vi "m2.vi"() -> ()   [LabVIEW 2016]
uses:
  <vilib>/rvi/interface/nirviOpenFPGA/nirviOpenFPGA.xnode
  <vilib>/rvi/interface/nirviMethod/nirviMethod.xnode
  <vilib>/FPGAPlugInAG/Dynamic/niLvFpga_Abort_Dynamic.vi
  <vilib>/FPGAPlugInAG/Dynamic/niLvFpga_Run_Dynamic.vi
  <vilib>/rvi/interface/nirviCloseFPGA/nirviCloseFPGA.xnode
  <vilib>/FPGAPlugInAG/Dynamic/niLvFpga_Reset_Dynamic.vi
  Common_RT_HealthAndStatus/RTHealthAndStatus/RTHealthAndStatus.lvclass
  MyHealthAndStatusReadFIFO/MyHealthAndStatusReadFIFO.lvclass
  MyHealthAndStatusWriteFIFO/MyHealthAndStatusWriteFIFO.lvclass
  Common_RT_Modbus/Modbus/Modbus.lvclass
  ModbusPort1ReadFIFO/ModbusPort1ReadFIFO.lvclass
  ModbusPort1WriteFIFO/ModbusPort1WriteFIFO.lvclass
  SoftwareControlledTrigger/SoftwareControlledTrigger.lvclass
  Common_RT_ILC/DataTypes/ILCSettings.ctl
  Common_RT_ILC/RTILC.lvlib
  Common_RT_ILC/ILC/ILC.lvclass
  <vilib>/rvi/interface/nirviMethod/StockFPGA_InlinedMethodWaitForSingleIRQ.vi
  <vilib>/FPGAPlugInAG/Dynamic/niLvFpga_WaitOnIrq_Dynamic.vi
  <vilib>/FPGAPlugInAG/Dynamic/niLvFpga_AcknowledgeIrq_Dynamic.vi
  Common_RT_Modbus/DynamicFrameParser/DynamicFrameParser.lvclass
  Common_RT_HPILC/HPILCFactory/HPILCFactory.lvclass
  Common_RT_HPILC/DataTypes/HPSettings.ctl
  Common_RT_HPILC/RTHPILC.lvlib
  Common_RT_HPILC/HPILC/HPILC.lvclass
  D:/Code/Common_RT_ILC/ILC/ILC.lvclass
  <vilib>/FPGAPlugInAG/Dynamic/niLvFpga_Close_Dynamic.vi
  FPGA Bitfiles/modbus1Port.lvbitx
  FPGA/main.vi
  <vilib>/FPGAPlugInAG/cRIO-9038/niLvFpga_Open_cRIO-9038.vi
  <vilib>/rvi/interface/common/dynamic/niFpgaDynamicAddResources.vi
  D:/Code/Common_RT_FPGA/IReadU32FIFO/IReadU32FIFO.lvclass
  D:/Code/Common_RT_FPGA/IReadU16FIFO/IReadU16FIFO.lvclass
  D:/Code/Common_RT_FPGA/IWriteU64FIFO/IWriteU64FIFO.lvclass
  D:/Code/Common_RT_FPGA/IWriteU16FIFO/IWriteU16FIFO.lvclass
  D:/Code/Common_RT_FPGA/IBooleanControl/IBooleanControl.lvclass
  Common_RT_ILC/DataTypes/ILCTelemetry.ctl
  Common_RT_Modbus/DataTypes/ExceptionCodes.ctl
  Common_RT_Modbus/RTModbus.lvlib
  Common_RT_ILC/DataTypes/ILCResponses.ctl
  Common_RT_HPILC/DataTypes/HPResponses.ctl
  Common_RT_HPILC/DataTypes/HPTelemetry.ctl
  Common_RT_ILC/DataTypes/ILCScanRates.ctl
panel:
  out "IRQ Timed Out 7":bool
  out "ParseSuccessful 7":bool
  in  "ForceAndStatus":bool
  out "HPTelemetry":T1
  out "HPResponses":T2 {"ForceAndStatus" items=["OK", "IllegalFunction", "IllegalDataAddress", "IllegalDataValue", "SlaveDeviceFailure", "Acknowledge", "SlaveDeviceBusy", "NegativeAcknowledge", "MemoryParityError", "GatewayPathUnavailable", "GatewayTargetDeviceFailedToRespond"]; "StepMotor" items=["OK", "IllegalFunction", "IllegalDataAddress", "IllegalDataValue", "SlaveDeviceFailure", "Acknowledge", "SlaveDeviceBusy", "NegativeAcknowledge", "MemoryParityError", "GatewayPathUnavailable", "GatewayTargetDeviceFailedToRespond"]}
  out "ParseSuccessful 6":bool
  out "IRQ Timed Out 6":bool
  in  "Steps":i8
  in  "StepMotor":bool
  in  "Boolean 2":bool
  in  "Boolean":bool
  out "IRQ Timed Out 5":bool
  out "ParseSuccessful 5":bool
  out "IRQ Timed Out 4":bool
  out "ParseSuccessful 4":bool
  out "IRQ Timed Out 3":bool
  out "ParseSuccessful 3":bool
  out "IRQ Timed Out 2":bool
  out "ParseSuccessful 2":bool
  out "ILCResponses":T4 {"ReadCalibration" items=["OK", "IllegalFunction", "IllegalDataAddress", "IllegalDataValue", "SlaveDeviceFailure", "Acknowledge", "SlaveDeviceBusy", "NegativeAcknowledge", "MemoryParityError", "GatewayPathUnavailable", "GatewayTargetDeviceFailedToRespond"]; "ReadDAC" items=["OK", "IllegalFunction", "IllegalDataAddress", "IllegalDataValue", "SlaveDeviceFailure", "Acknowledge", "SlaveDeviceBusy", "NegativeAcknowledge", "MemoryParityError", "GatewayPathUnavailable", "GatewayTargetDeviceFailedToRespond"]; "ADCOffsetSensitivity" items=["OK", "IllegalFunction", "IllegalDataAddress", "IllegalDataValue", "SlaveDeviceFailure", "Acknowledge", "SlaveDeviceBusy", "NegativeAcknowledge", "MemoryParityError", "GatewayPathUnavailable", "GatewayTargetDeviceFailedToRespond"]; "ADCScanRate" items=["OK", "IllegalFunction", "IllegalDataAddress", "IllegalDataValue", "SlaveDeviceFailure", "Acknowledge", "SlaveDeviceBusy", "NegativeAcknowledge", "MemoryParityError", "GatewayPathUnavailable", "GatewayTargetDeviceFailedToRespond"]; "Reset" items=["OK", "IllegalFunction", "IllegalDataAddress", "IllegalDataValue", "SlaveDeviceFailure", "Acknowledge", "SlaveDeviceBusy", "NegativeAcknowledge", "MemoryParityError", "GatewayPathUnavailable", "GatewayTargetDeviceFailedToRespond"]; "SetTemporaryAddress" items=["OK", "IllegalFunction", "IllegalDataAddress", "IllegalDataValue", "SlaveDeviceFailure", "Acknowledge", "SlaveDeviceBusy", "NegativeAcknowledge", "MemoryParityError", "GatewayPathUnavailable", "GatewayTargetDeviceFailedToRespond"]; "ILCMode" items=["OK", "IllegalFunction", "IllegalDataAddress", "IllegalDataValue", "SlaveDeviceFailure", "Acknowledge", "SlaveDeviceBusy", "NegativeAcknowledge", "MemoryParityError", "GatewayPathUnavailable", "GatewayTargetDeviceFailedToRespond"]; "ReportServerStatus" items=["OK", "IllegalFunction", "IllegalDataAddress", "IllegalDataValue", "SlaveDeviceFailure", "Acknowledge", "SlaveDeviceBusy", "NegativeAcknowledge", "MemoryParityError", "GatewayPathUnavailable", "GatewayTargetDeviceFailedToRespond"]; "ReportServerID" items=["OK", "IllegalFunction", "IllegalDataAddress", "IllegalDataValue", "SlaveDeviceFailure", "Acknowledge", "SlaveDeviceBusy", "NegativeAcknowledge", "MemoryParityError", "GatewayPathUnavailable", "GatewayTargetDeviceFailedToRespond"]}
  out "ParseSuccessful":bool
  out "IRQ Timed Out":bool
  out "ILCTelemetry":T5 {"ADCScanRate" items=["50 Hz"=0, "60 Hz"=1, "100 Hz"=2, "120 Hz"=3, "200 Hz"=4, "240 Hz"=5, "300 Hz"=6, "400 Hz"=7, "480 Hz"=8, "600 Hz"=9, "1200 Hz"=10, "2400 Hz"=11, "4800 Hz"=12, "No Change"=255]}
  in  "SetTemporaryAddress":bool
  in  "Reset":bool
  in  "ReportServerStatus":bool
  in  "ReportServerID":bool
  in  "TemporaryAddress":u8
  in  "ILCMode":u16
  in  "SetILCMode":bool
  out "Port 1 Status Bits":u64 format="%016b"
  out "error out":errorcluster
  out "Port 1 Frames Received":i64
  out "Port 1 Bytes Received":i64
  out "Port 1 Frames Transmitted":i64
  out "Port 1 Bytes Transmitted":i64
  # "Port 1 = Modbus"
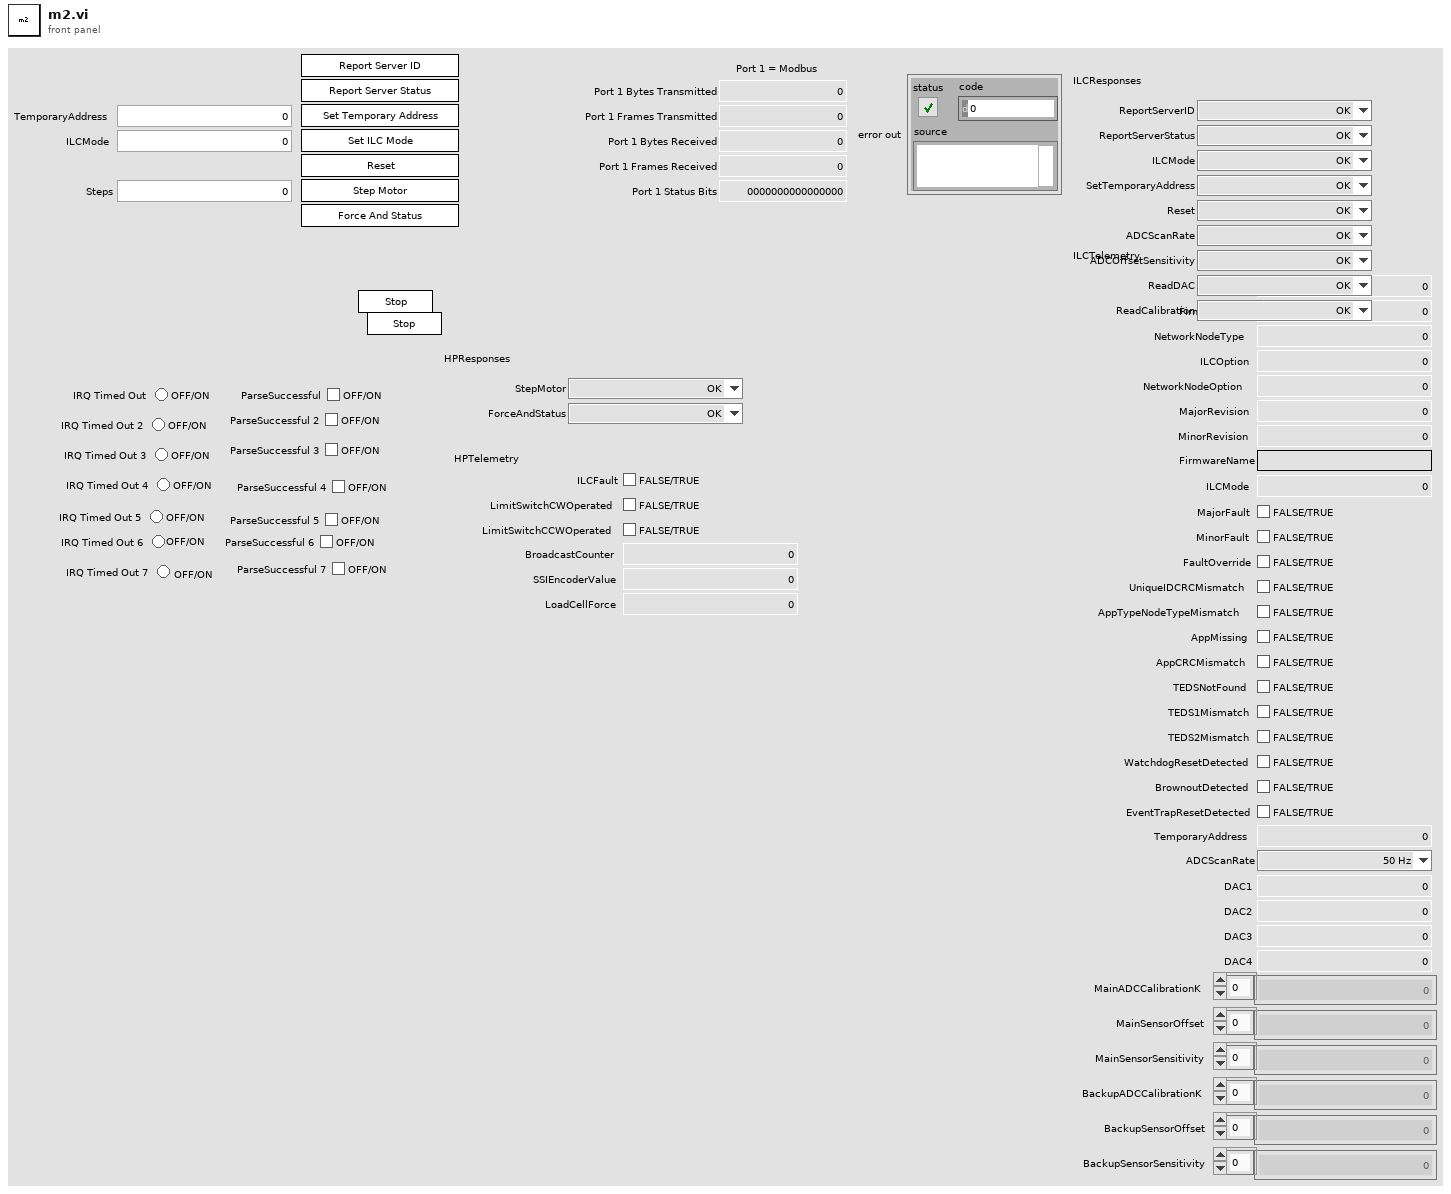
[diagram p1: front panel]
types:
  T1 = typedef "RTHPILC.lvlib/HPTelemetry.ctl" = cluster{"ILCFault":bool, "LimitSwitchCWOperated":bool, "LimitSwitchCCWOperated":bool, "BroadcastCounter":u8, "SSIEncoderValue":i32, "LoadCellForce":sgl}
  T2 = typedef "RTHPILC.lvlib/HPResponses.ctl" = cluster{"StepMotor":T3, "ForceAndStatus":T3}
  T3 = typedef "RTModbus.lvlib/ExceptionCodes.ctl" = u16
  T4 = typedef "RTILC.lvlib/ILCResponses.ctl" = cluster{"ReportServerID":T3, "ReportServerStatus":T3, "ILCMode":T3, "SetTemporaryAddress":T3, "Reset":T3, "ADCScanRate":T3, "ADCOffsetSensitivity":T3, "ReadDAC":T3, "ReadCalibration":T3}
  T5 = typedef "RTILC.lvlib/ILCTelemetry.ctl" = cluster{"UniqueID":u64, "FirmwareType":u8, "NetworkNodeType":u8, "ILCOption":u8, "NetworkNodeOption":u8, "MajorRevision":u8, "MinorRevision":u8, "FirmwareName":string, "ILCMode":u16, "MajorFault":bool, "MinorFault":bool, "FaultOverride":bool, "UniqueIDCRCMismatch":bool, "AppTypeNodeTypeMismatch":bool, "AppMissing":bool, "AppCRCMismatch":bool, "TEDSNotFound":bool, "TEDS1Mismatch":bool, "TEDS2Mismatch":bool, "WatchdogResetDetected":bool, "BrownoutDetected":bool, "EventTrapResetDetected":bool, "TemporaryAddress":u8, "ADCScanRate":T6, "DAC1":u16, "DAC2":u16, "DAC3":u16, "DAC4":u16, "MainADCCalibrationK":sgl[], "MainSensorOffset":sgl[], "MainSensorSensitivity":sgl[], "BackupADCCalibrationK":sgl[], "BackupSensorOffset":sgl[], "BackupSensorSensitivity":sgl[]}
  T6 = typedef "RTILC.lvlib/ILCScanRates.ctl" = u8
  T7 = typedef "RTHPILC.lvlib/HPSettings.ctl" = cluster{"ILCSettings":T8, "ID":i16, "ReferencePosition":i32}
  T8 = typedef "RTILC.lvlib/ILCSettings.ctl" = cluster{"Subnet":u8, "Address":u8}
  T9 = typedef "RTModbus.lvlib/Frame.ctl" = cluster{"Data":u8[], "WaitForTrigger":bool, "WaitForRx":u16, "TriggerIRQ":bool, "DelayTicks":u16, "DelayMicroseconds":u16, "DelayMilliseconds":u16}
  T10 = typedef "RTILC.lvlib/ILCData.ctl" = cluster{"Constants":T11, "Command":T12, "Telemetry":T5, "Responses":T4, "Timings":T13}
  T11 = typedef "RTILC.lvlib/ILCConstants.ctl" = cluster{"Subnet":u8, "Address":u8}
  T12 = typedef "RTILC.lvlib/ILCCommand.ctl" = cluster{"ILCMode":u16, "TemporaryAddress":u8, "ADCScanRate":T6, "ADCChannel":u8, "ADCOffset":sgl, "ADCSensitivity":sgl}
  T13 = typedef "RTILC.lvlib/ILCTimings.ctl" = cluster{"ADCOffsetSensitivity":u32, "ADCScanRate":u32, "ILCMode":u32, "ReadCalibration":u32, "ReportServerID":u32, "ReportServerStatus":u32, "Reset":u32, "SetTemporaryAddress":u32}
  T14 = typedef "RTHPILC.lvlib/HPData.ctl" = cluster{"Constants":T15, "Command":T16, "Telemetry":T1, "Responses":T2, "Timings":T17}
  T15 = typedef "RTHPILC.lvlib/HPConstants.ctl" = cluster{"ID":i16, "ReferencePosition":i32}
  T16 = typedef "RTHPILC.lvlib/HPCommand.ctl" = cluster{"Steps":i8}
  T17 = typedef "RTHPILC.lvlib/HPTimings.ctl" = cluster{"BroadcastStepMotor":u32, "ForceAndStatus":u32, "FreezeSensorValues":u32, "StepMotor":u32}
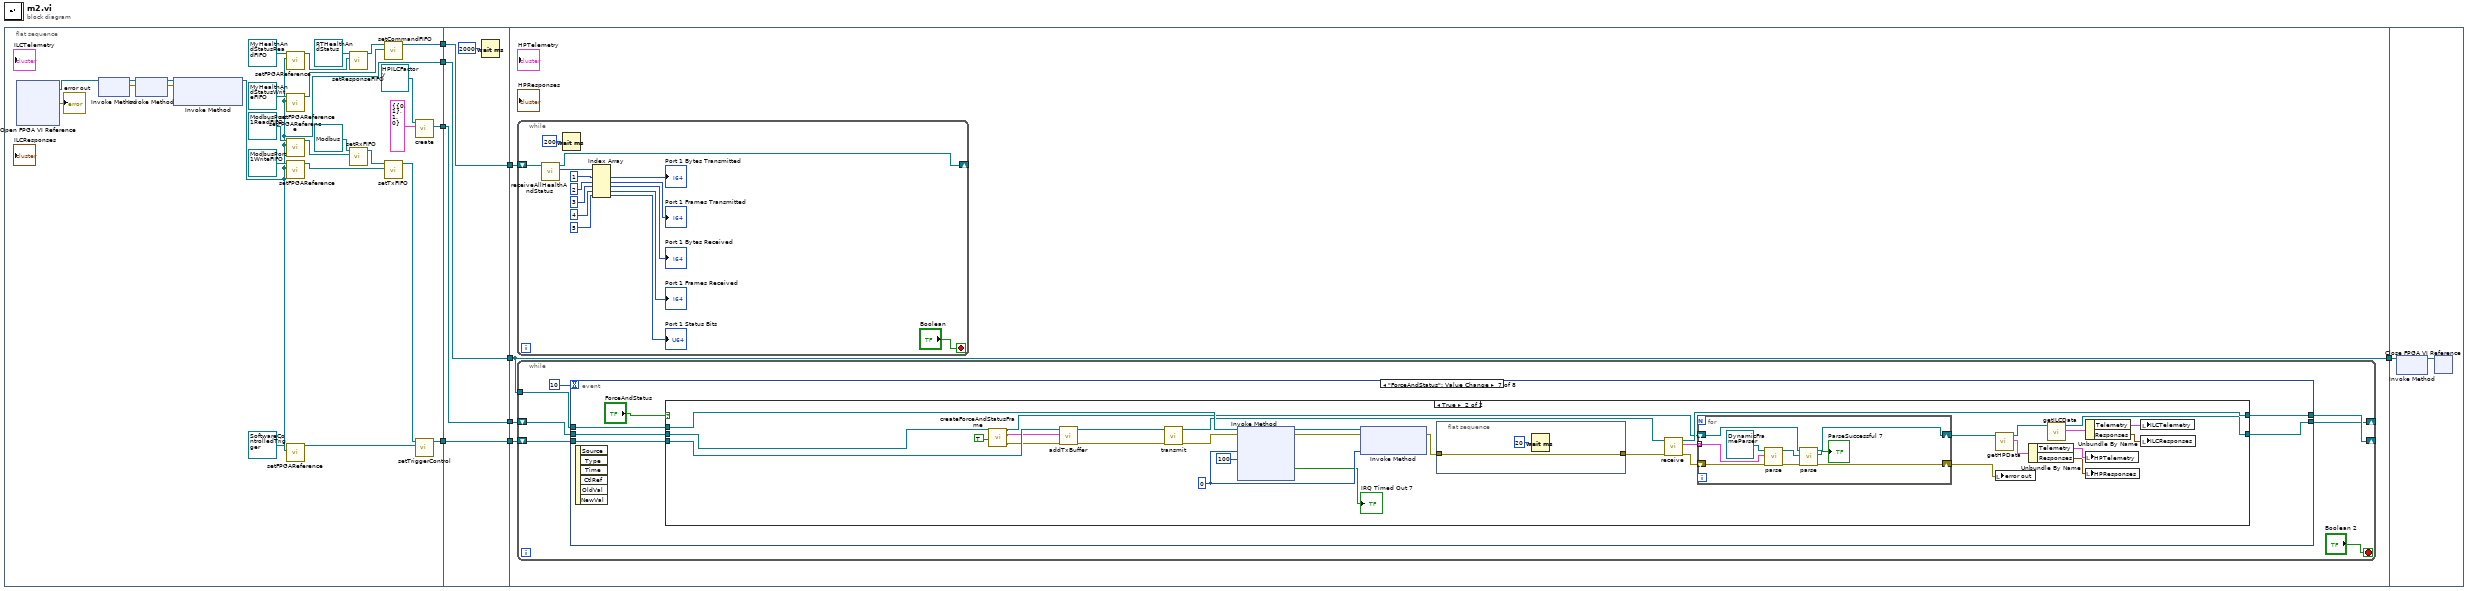
[diagram p0: block diagram]
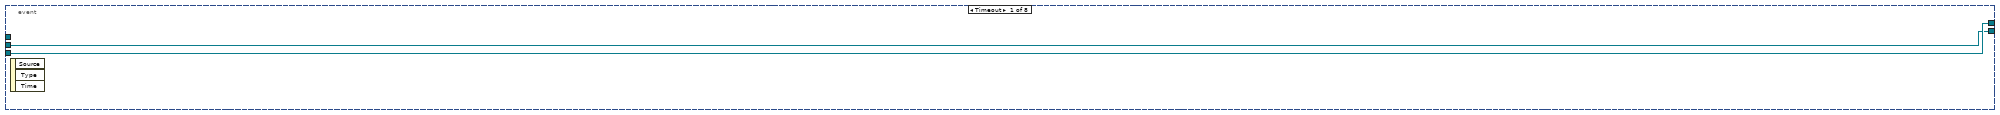
[diagram p2: hidden frame]
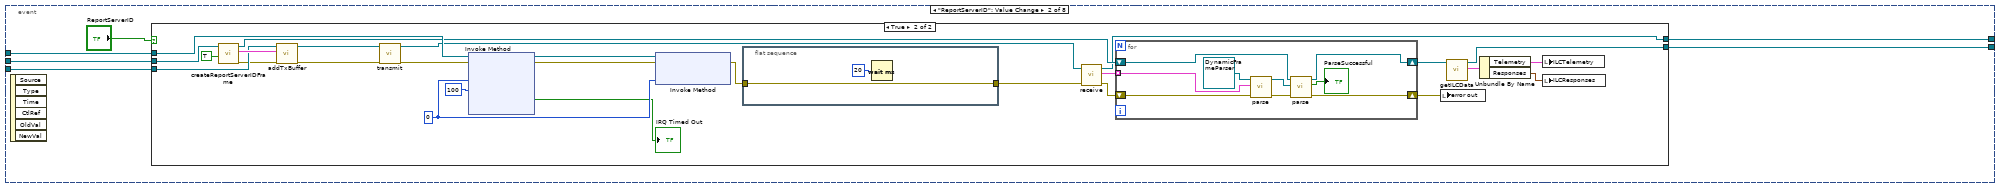
[diagram p3: hidden frame]
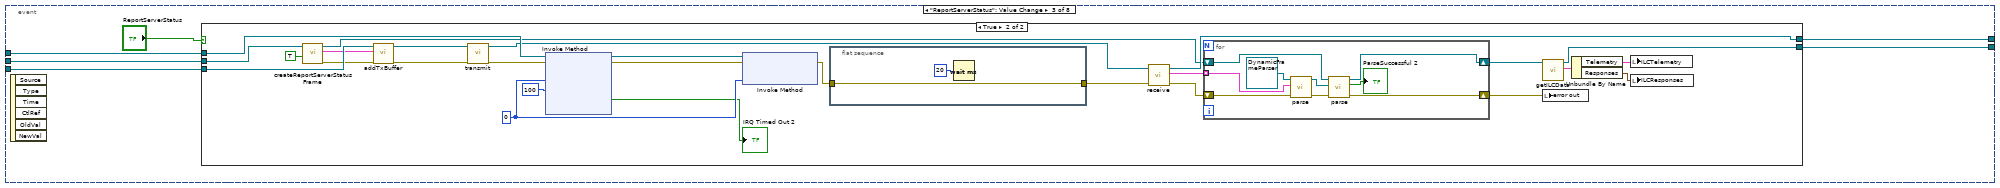
[diagram p5: hidden frame]
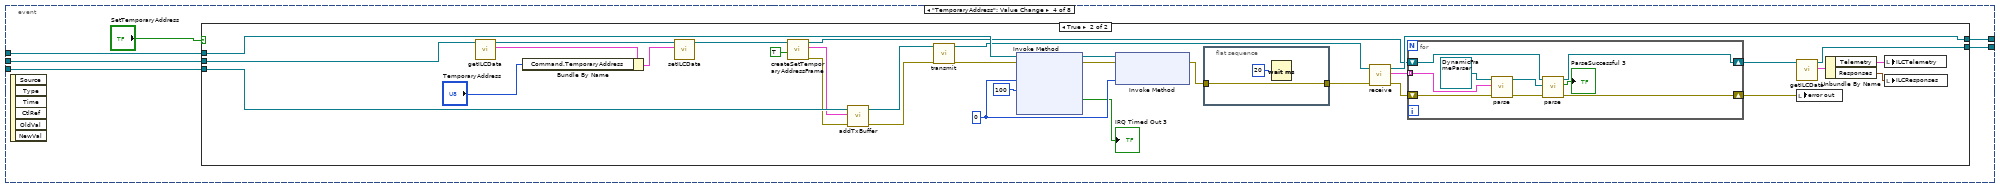
[diagram p7: hidden frame]
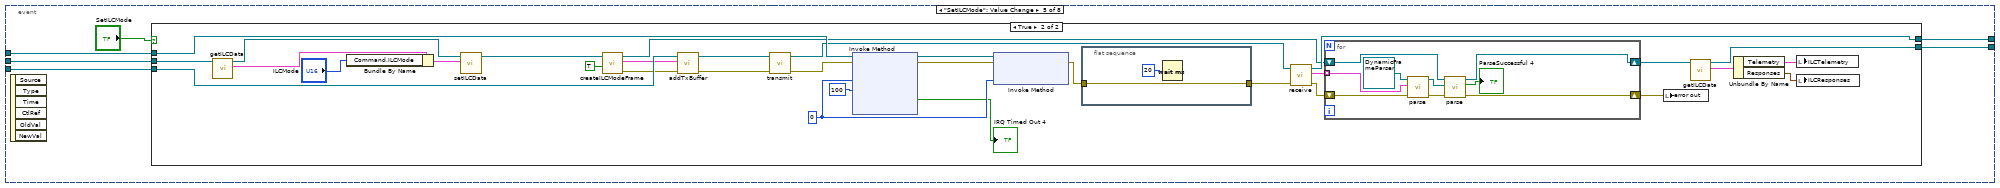
[diagram p9: hidden frame]
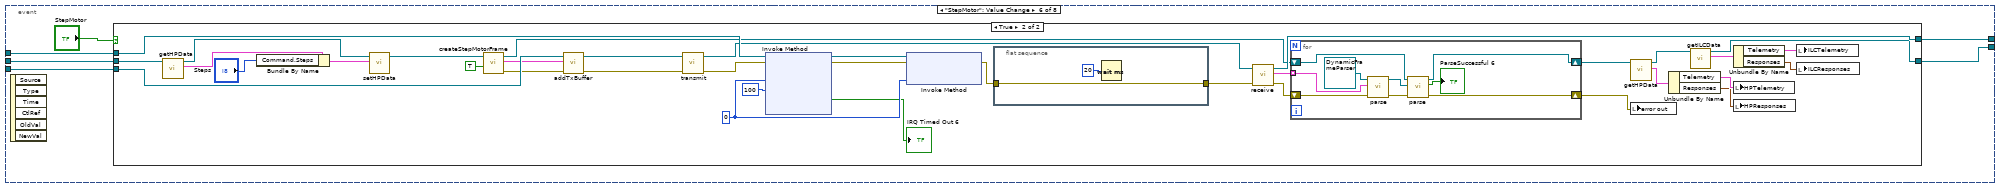
[diagram p11: hidden frame]
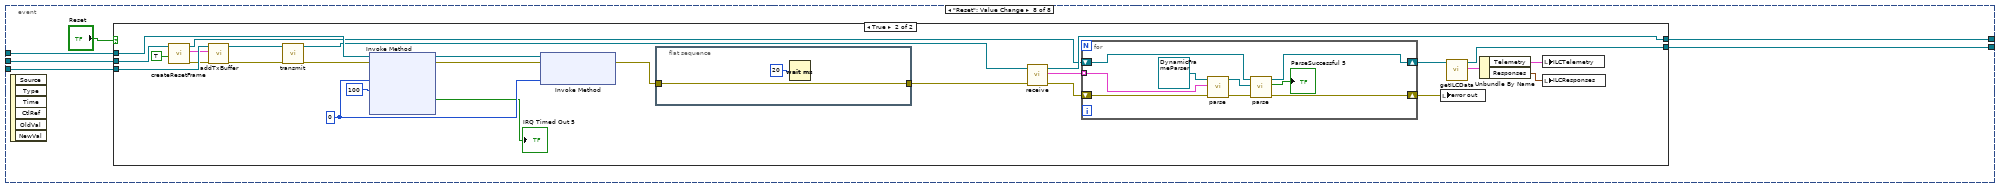
[diagram p14: hidden frame]
diagram:
  n1 = flat-sequence {
    tunnel: [w17] -> w9
    tunnel: [w14] -> w6
    tunnel: [w32] -> w4
    tunnel: [w10] -> w1
    tunnel: w9 -> [w41]
    tunnel: [w41] -> w8
    tunnel: w6 -> [w39]
    tunnel: [w39] -> w5
    tunnel: w4 -> [w38]
    tunnel: [w38] -> w3
    tunnel: [w37] -> w2
    tunnel: w1 -> [w37]
    tunnel: w8 -> [w42]
    tunnel: [w42] -> w7
    tunnel: w5 -> [w45]
    tunnel: w3 -> [w44]
    tunnel: w2 -> [w43]
    tunnel: w7 -> [w415]
    frame #0 {
      n2 = xnode "Open FPGA VI Reference"() -> ("FPGA VI Reference Out"=w19:refnum<k20>, "error out"=→"error out":errorcluster)  [unwired: 2 in]
      n3 = xnode "Invoke Method"("FPGA VI Reference In"=w19) -> ("FPGA VI Reference Out"=w36:refnum<k20>, "error out"=w21:errorcluster)  [unwired: 1 in]
      n4 = xnode "Invoke Method"("FPGA VI Reference In"=w36, "error in"=w21) -> ("FPGA VI Reference Out"=w35:refnum<k20>, "error out"=w20:errorcluster)
      n5 = xnode "Invoke Method"("FPGA VI Reference In"=w35, "error in"=w20) -> ("FPGA VI Reference Out"=w17:refnum<k20>)  [unwired: 1 in, 1 out]
      n6 = call "setFPGAReference.vi"("FPGAReference"=w17, "MyHealthAndStatusReadFIFO in"=refnum<class "MyHealthAndStatusReadFIFO.lvclass"> refnum ("MyHealthAndStatusReadFIFO.lvclass")) -> ("MyHealthAndStatusReadFIFO out"=w28:refnum<class "MyHealthAndStatusReadFIFO.lvclass">)  [unwired: 9 in]
      n7 = call "setFPGAReference.vi"("FPGAReference"=w17, "MyHealthAndStatusWriteFIFO in"=refnum<class "MyHealthAndStatusWriteFIFO.lvclass"> refnum ("MyHealthAndStatusWriteFIFO.lvclass")) -> ("MyHealthAndStatusWriteFIFO out"=w26:refnum<class "MyHealthAndStatusWriteFIFO.lvclass">)  [unwired: 9 in]
      n8 = call "setFPGAReference.vi"("FPGAReference"=w17, "ModbusPort1ReadFIFO in"=refnum<class "ModbusPort1ReadFIFO.lvclass"> refnum ("ModbusPort1ReadFIFO.lvclass")) -> ("ModbusPort1ReadFIFO out"=w24:refnum<class "ModbusPort1ReadFIFO.lvclass">)  [unwired: 9 in]
      n9 = call "setFPGAReference.vi"("FPGAReference"=w17, "ModbusPort1WriteFIFO in"=refnum<class "ModbusPort1WriteFIFO.lvclass"> refnum ("ModbusPort1WriteFIFO.lvclass")) -> ("ModbusPort1WriteFIFO out"=w22:refnum<class "ModbusPort1WriteFIFO.lvclass">)  [unwired: 9 in]
      n10 = call "setFPGAReference.vi"("FPGAReference"=w17, "SoftwareControlledTrigger in"=refnum<class "SoftwareControlledTrigger.lvclass"> refnum ("SoftwareControlledTrigger.lvclass")) -> ("SoftwareControlledTrigger out"=w13:refnum<class "SoftwareControlledTrigger.lvclass">)  [unwired: 9 in]
      n11 = call "setResponseFIFO.vi"("ReadU32FIFO"=w28, "RTHealthAndStatus in"=refnum<class "RTHealthAndStatus.lvclass"> refnum ("RTHealthAndStatus.lvlib:RTHealthAndStatus.lvclass")) -> ("RTHealthAndStatus out"=w33:refnum<class "RTHealthAndStatus.lvclass">)  [unwired: 9 in]
      n12 = call "setRxFIFO.vi"("ReadU16FIFO"=w24, "Modbus in"=refnum<class "Modbus.lvclass"> refnum ("RTModbus.lvlib:Modbus.lvclass")) -> ("Modbus out"=w30:refnum<class "Modbus.lvclass">)  [unwired: 9 in]
      n13 = call "setCommandFIFO.vi"("WriteU64FIFO"=w26, "RTHealthAndStatus in"=w33) -> ("RTHealthAndStatus out"=w32:refnum<class "RTHealthAndStatus.lvclass">)  [unwired: 9 in]
      n14 = call "setTxFIFO.vi"("WriteU16FIFO"=w22, "Modbus in"=w30) -> ("Modbus out"=w15:refnum<class "Modbus.lvclass">)  [unwired: 9 in]
      n15 = call "create.vi"("HPSettings"=T7 {"ILCSettings"={"Subnet"=0, "Address"=1}, "ID"=1, "ReferencePosition"=0}, "HardPointActuatorFactory in"=refnum<class "HPILCFactory.lvclass"> refnum ("RTHPILC.lvlib:HPILCFactory.lvclass")) -> ("HardPointActuator"=w10:refnum<class "HPILC.lvclass">)  [unwired: 7 in, 2 out]
      n16 = call "setTriggerControl.vi"("BooleanControl"=w13, "Modbus in"=w15) -> ("Modbus out"=w14:refnum<class "Modbus.lvclass">)  [unwired: 9 in]
    }
    frame #1 {
      n17 = Wait (ms)(milliseconds to wait=u32 2000) -> ()  [unwired: 1 out]
    }
    frame #2 {
      n18 = while {
        shift-right: [w58] -> _
        shift-left: w44 -> [w59]
        stop <- "Boolean" stop-if-true
        n19 = call "receiveAllHealthAndStatus.vi"("RTHealthAndStatus in"=w59) -> ("Data"=w53:u32[], "RTHealthAndStatus out"=w58:refnum<class "RTHealthAndStatus.lvclass">)  [unwired: 8 in, 1 out]
        n20 = Wait (ms)(milliseconds to wait=u32 200) -> ()  [unwired: 1 out]
        n21 = Index Array(array=w53, index #1=1 ("index"), index #2=2 ("index"), index #3=3 ("index"), index #4=4 ("index"), index #5=5 ("index")) -> (element #1=→"Port 1 Bytes Transmitted":u32, element #2=→"Port 1 Frames Transmitted":u32, element #3=→"Port 1 Bytes Received":u32, element #4=→"Port 1 Frames Received":u32, element #5=→"Port 1 Status Bits":u32)
      }
      n22 = while {
        shift-right: [w65] -> _
        shift-left: w45 -> [w66]
        shift-right: [w63] -> _
        shift-left: w43 -> [w64]
        tunnel: w42 -> [w62]
        stop <- "Boolean 2" stop-if-true
        n23 = event shown="[6] \"ForceAndStatus\": Value Change" {
          selector: _ -> [_ _ _ _ _ _ _ _]
          dyn-events: _ -> [_ _ _ _ _ _ _ _]
          timeout: 10 -> [_ _ _ _ _ _ _ _]
          tunnel: w66 -> [w69 w73 w120 w166 w217 w268 w323 w373]
          tunnel: [w69 w71 w118 w164 w215 w266 w321 w371] -> w65
          tunnel: w64 -> [w68 w74 w121 w167 w218 w269 w324 w374]
          tunnel: [w68 w72 w119 w165 w216 w267 w322 w372] -> w63
          tunnel: w62 -> [_ w70 w117 w163 w214 w265 w320 w370]
          event Timeout {
            n24 = event-data() -> ()  [unwired: 1 in, 3 out]
          }
          event "ReportServerID": Value Change {
            n25 = event-data() -> ()  [unwired: 1 in, 6 out]
            n26 = case shown="True" "ReportServerID" {
              tunnel: w74 -> [w77 w104]
              tunnel: w73 -> [w76 w102]
              tunnel: [w77 w81] -> w72
              tunnel: [w76 w84] -> w71
              tunnel: w70 -> [_ w98]
              frame False {
              }
              frame True {
                w96 = 0 ("IRQ Number(s)")
                n27 = call "createReportServerIDFrame.vi"("TriggerIRQ"=TRUE, "ILC in"=w104) -> ("error out"=w100:errorcluster, "Frame"=w103:T9, "ILC out"=w87:refnum<class "HPILC.lvclass">)  [unwired: 7 in]
                n28 = call-dynamic "addTxBuffer.vi"("error in (no error)"=w100, "Frame"=w103, "Modbus in"=w102) -> ("error out"=w99:errorcluster, "Modbus out"=w101:refnum<class "Modbus.lvclass">)  [unwired: 7 in]
                n29 = call-dynamic "transmit.vi"("error in (no error)"=w99, "Modbus in"=w101) -> ("error out"=w92:errorcluster, "Modbus out"=w85:refnum<class "Modbus.lvclass">)  [unwired: 8 in]
                n30 = xnode "Invoke Method"("FPGA VI Reference In"=w98, "error in"=w92, "IRQ Number(s)"=w96, "Timeout (ms)"=100) -> ("FPGA VI Reference Out"=w97:refnum<k20>, "error out"=w93:errorcluster, "Timed Out"=→"IRQ Timed Out":bool)  [unwired: 1 out]
                n31 = xnode "Invoke Method"("FPGA VI Reference In"=w97, "error in"=w93, "IRQ Number(s)"=w96) -> ("error out"=w90:errorcluster)  [unwired: 1 out]
                n32 = flat-sequence {
                  tunnel: w90 -> [w114]
                  tunnel: [w114] -> w89
                  frame #0 {
                    n33 = Wait (ms)(milliseconds to wait=u32 20) -> ()  [unwired: 1 out]
                  }
                }
                n34 = call-dynamic "receive.vi"("error in (no error)"=w89, "Modbus in"=w85) -> ("error out"=w86:errorcluster, "Data"=w88:T9[], "Modbus out"=w84:refnum<class "Modbus.lvclass">)  [unwired: 7 in]
                n35 = for {
                  tunnel: w88 -> [w112] mode=indexing
                  shift-right: [w109] -> w82
                  shift-left: w87 -> [w110]
                  shift-right: [w106] -> w83
                  shift-left: w86 -> [w108]
                  n36 = call "parse.vi"("error in (no error)"=w108, "Frame"=w112, "FrameParser in"=refnum<class "DynamicFrameParser.lvclass"> refnum ("RTModbus.lvlib:DynamicFrameParser.lvclass")) -> ("error out"=w107:errorcluster, "FrameParser out"=w111:refnum<class "DynamicFrameParser.lvclass">)  [unwired: 7 in]
                  n37 = call-dynamic "parse.vi"("error in (no error)"=w107, "DynamicFrameParser"=w111, "HPILC in"=w110) -> ("error out"=w106:errorcluster, "ParseSuccessful"=→"ParseSuccessful":bool, "HPILC out"=w109:refnum<class "HPILC.lvclass">)  [unwired: 6 in]
                }
                n38 = local write "error out"(w83) -> ()
                n39 = call "getILCData.vi"("ILC in"=w82) -> ("ILCData"=w80:T10, "ILC out"=w81:refnum<class "HPILC.lvclass">)  [unwired: 9 in]
                n40 = Unbundle By Name(w80) -> ("Telemetry"=w79:T5, "Responses"=w78:T4)
                n41 = local write "ILCTelemetry"(w79) -> ()
                n42 = local write "ILCResponses"(w78) -> ()
              }
            }
          }
          event "ReportServerStatus": Value Change {
            n43 = event-data() -> ()  [unwired: 1 in, 6 out]
            n44 = case shown="True" "ReportServerStatus" {
              tunnel: w121 -> [w123 w128]
              tunnel: w120 -> [w122 w150]
              tunnel: [w123 w132] -> w119
              tunnel: [w122 w135] -> w118
              tunnel: w117 -> [_ w147]
              frame False {
              }
              frame True {
                w145 = 0 ("IRQ Number(s)")
                n45 = call "createReportServerStatusFrame.vi"("TriggerIRQ"=TRUE, "ILC in"=w128) -> ("error out"=w124:errorcluster, "Frame"=w126:T9, "ILC out"=w125:refnum<class "HPILC.lvclass">)  [unwired: 7 in]
                n46 = call-dynamic "addTxBuffer.vi"("error in (no error)"=w124, "Frame"=w126, "Modbus in"=w150) -> ("error out"=w148:errorcluster, "Modbus out"=w149:refnum<class "Modbus.lvclass">)  [unwired: 7 in]
                n47 = call-dynamic "transmit.vi"("error in (no error)"=w148, "Modbus in"=w149) -> ("error out"=w141:errorcluster, "Modbus out"=w136:refnum<class "Modbus.lvclass">)  [unwired: 8 in]
                n48 = xnode "Invoke Method"("FPGA VI Reference In"=w147, "error in"=w141, "IRQ Number(s)"=w145, "Timeout (ms)"=100) -> ("FPGA VI Reference Out"=w146:refnum<k20>, "error out"=w142:errorcluster, "Timed Out"=→"IRQ Timed Out 2":bool)  [unwired: 1 out]
                n49 = xnode "Invoke Method"("FPGA VI Reference In"=w146, "error in"=w142, "IRQ Number(s)"=w145) -> ("error out"=w140:errorcluster)  [unwired: 1 out]
                n50 = flat-sequence {
                  tunnel: w140 -> [w160]
                  tunnel: [w160] -> w139
                  frame #0 {
                    n51 = Wait (ms)(milliseconds to wait=u32 20) -> ()  [unwired: 1 out]
                  }
                }
                n52 = call-dynamic "receive.vi"("error in (no error)"=w139, "Modbus in"=w136) -> ("error out"=w137:errorcluster, "Data"=w138:T9[], "Modbus out"=w135:refnum<class "Modbus.lvclass">)  [unwired: 7 in]
                n53 = for {
                  tunnel: w138 -> [w158] mode=indexing
                  shift-right: [w155] -> w133
                  shift-left: w125 -> [w156]
                  shift-right: [w152] -> w134
                  shift-left: w137 -> [w154]
                  n54 = call "parse.vi"("error in (no error)"=w154, "Frame"=w158, "FrameParser in"=refnum<class "DynamicFrameParser.lvclass"> refnum ("RTModbus.lvlib:DynamicFrameParser.lvclass")) -> ("error out"=w153:errorcluster, "FrameParser out"=w157:refnum<class "DynamicFrameParser.lvclass">)  [unwired: 7 in]
                  n55 = call-dynamic "parse.vi"("error in (no error)"=w153, "DynamicFrameParser"=w157, "HPILC in"=w156) -> ("error out"=w152:errorcluster, "ParseSuccessful"=→"ParseSuccessful 2":bool, "HPILC out"=w155:refnum<class "HPILC.lvclass">)  [unwired: 6 in]
                }
                n56 = call "getILCData.vi"("ILC in"=w133) -> ("ILCData"=w131:T10, "ILC out"=w132:refnum<class "HPILC.lvclass">)  [unwired: 9 in]
                n57 = local write "error out"(w134) -> ()
                n58 = Unbundle By Name(w131) -> ("Telemetry"=w130:T5, "Responses"=w129:T4)
                n59 = local write "ILCTelemetry"(w130) -> ()
                n60 = local write "ILCResponses"(w129) -> ()
              }
            }
          }
          event "TemporaryAddress": Value Change {
            n61 = event-data() -> ()  [unwired: 1 in, 6 out]
            n62 = case shown="True" "SetTemporaryAddress" {
              tunnel: w167 -> [w169 w175]
              tunnel: w166 -> [w168 w201]
              tunnel: [w169 w183] -> w165
              tunnel: [w168 w186] -> w164
              tunnel: w163 -> [_ w198]
              frame False {
              }
              frame True {
                w196 = 0 ("IRQ Number(s)")
                n63 = call "getILCData.vi"("ILC in"=w175) -> ("ILCData"=w174:T10, "ILC out"=w172:refnum<class "HPILC.lvclass">)  [unwired: 9 in]
                n64 = Bundle By Name(cluster=w174, "Command.TemporaryAddress"="TemporaryAddress") -> (w173:T10)
                n65 = call "setILCData.vi"("ILCData"=w173, "ILC in"=w172) -> ("ILC out"=w171:refnum<class "HPILC.lvclass">)  [unwired: 9 in]
                n66 = call "createSetTemporaryAddressFrame.vi"("TriggerIRQ"=TRUE, "ILC in"=w171) -> ("error out"=w177:errorcluster, "Frame"=w178:T9, "ILC out"=w179:refnum<class "HPILC.lvclass">)  [unwired: 7 in]
                n67 = call-dynamic "addTxBuffer.vi"("error in (no error)"=w177, "Frame"=w178, "Modbus in"=w201) -> ("error out"=w199:errorcluster, "Modbus out"=w200:refnum<class "Modbus.lvclass">)  [unwired: 7 in]
                n68 = call-dynamic "transmit.vi"("error in (no error)"=w199, "Modbus in"=w200) -> ("error out"=w192:errorcluster, "Modbus out"=w187:refnum<class "Modbus.lvclass">)  [unwired: 8 in]
                n69 = xnode "Invoke Method"("FPGA VI Reference In"=w198, "error in"=w192, "IRQ Number(s)"=w196, "Timeout (ms)"=100) -> ("FPGA VI Reference Out"=w197:refnum<k20>, "error out"=w193:errorcluster, "Timed Out"=→"IRQ Timed Out 3":bool)  [unwired: 1 out]
                n70 = xnode "Invoke Method"("FPGA VI Reference In"=w197, "error in"=w193, "IRQ Number(s)"=w196) -> ("error out"=w191:errorcluster)  [unwired: 1 out]
                n71 = flat-sequence {
                  tunnel: w191 -> [w211]
                  tunnel: [w211] -> w190
                  frame #0 {
                    n72 = Wait (ms)(milliseconds to wait=u32 20) -> ()  [unwired: 1 out]
                  }
                }
                n73 = call-dynamic "receive.vi"("error in (no error)"=w190, "Modbus in"=w187) -> ("error out"=w188:errorcluster, "Data"=w189:T9[], "Modbus out"=w186:refnum<class "Modbus.lvclass">)  [unwired: 7 in]
                n74 = for {
                  tunnel: w189 -> [w209] mode=indexing
                  shift-right: [w206] -> w184
                  shift-left: w179 -> [w207]
                  shift-right: [w203] -> w185
                  shift-left: w188 -> [w205]
                  n75 = call "parse.vi"("error in (no error)"=w205, "Frame"=w209, "FrameParser in"=refnum<class "DynamicFrameParser.lvclass"> refnum ("RTModbus.lvlib:DynamicFrameParser.lvclass")) -> ("error out"=w204:errorcluster, "FrameParser out"=w208:refnum<class "DynamicFrameParser.lvclass">)  [unwired: 7 in]
                  n76 = call-dynamic "parse.vi"("error in (no error)"=w204, "DynamicFrameParser"=w208, "HPILC in"=w207) -> ("error out"=w203:errorcluster, "ParseSuccessful"=→"ParseSuccessful 3":bool, "HPILC out"=w206:refnum<class "HPILC.lvclass">)  [unwired: 6 in]
                }
                n77 = call "getILCData.vi"("ILC in"=w184) -> ("ILCData"=w182:T10, "ILC out"=w183:refnum<class "HPILC.lvclass">)  [unwired: 9 in]
                n78 = local write "error out"(w185) -> ()
                n79 = Unbundle By Name(w182) -> ("Telemetry"=w181:T5, "Responses"=w180:T4)
                n80 = local write "ILCTelemetry"(w181) -> ()
                n81 = local write "ILCResponses"(w180) -> ()
              }
            }
          }
          event "SetILCMode": Value Change {
            n82 = event-data() -> ()  [unwired: 1 in, 6 out]
            n83 = case shown="True" "SetILCMode" {
              tunnel: w218 -> [w220 w230]
              tunnel: w217 -> [w219 w252]
              tunnel: [w220 w234] -> w216
              tunnel: [w219 w237] -> w215
              tunnel: w214 -> [_ w249]
              frame False {
              }
              frame True {
                w247 = 0 ("IRQ Number(s)")
                n84 = call "getILCData.vi"("ILC in"=w230) -> ("ILCData"=w229:T10, "ILC out"=w227:refnum<class "HPILC.lvclass">)  [unwired: 9 in]
                n85 = Bundle By Name(cluster=w229, "Command.ILCMode"="ILCMode") -> (w228:T10)
                n86 = call "setILCData.vi"("ILCData"=w228, "ILC in"=w227) -> ("ILC out"=w225:refnum<class "HPILC.lvclass">)  [unwired: 9 in]
                n87 = call "createILCModeFrame.vi"("TriggerIRQ"=TRUE, "ILC in"=w225) -> ("error out"=w221:errorcluster, "Frame"=w223:T9, "ILC out"=w222:refnum<class "HPILC.lvclass">)  [unwired: 7 in]
                n88 = call-dynamic "addTxBuffer.vi"("error in (no error)"=w221, "Frame"=w223, "Modbus in"=w252) -> ("error out"=w250:errorcluster, "Modbus out"=w251:refnum<class "Modbus.lvclass">)  [unwired: 7 in]
                n89 = call-dynamic "transmit.vi"("error in (no error)"=w250, "Modbus in"=w251) -> ("error out"=w243:errorcluster, "Modbus out"=w238:refnum<class "Modbus.lvclass">)  [unwired: 8 in]
                n90 = xnode "Invoke Method"("FPGA VI Reference In"=w249, "error in"=w243, "IRQ Number(s)"=w247, "Timeout (ms)"=100) -> ("FPGA VI Reference Out"=w248:refnum<k20>, "error out"=w244:errorcluster, "Timed Out"=→"IRQ Timed Out 4":bool)  [unwired: 1 out]
                n91 = xnode "Invoke Method"("FPGA VI Reference In"=w248, "error in"=w244, "IRQ Number(s)"=w247) -> ("error out"=w242:errorcluster)  [unwired: 1 out]
                n92 = flat-sequence {
                  tunnel: w242 -> [w262]
                  tunnel: [w262] -> w241
                  frame #0 {
                    n93 = Wait (ms)(milliseconds to wait=u32 20) -> ()  [unwired: 1 out]
                  }
                }
                n94 = call-dynamic "receive.vi"("error in (no error)"=w241, "Modbus in"=w238) -> ("error out"=w239:errorcluster, "Data"=w240:T9[], "Modbus out"=w237:refnum<class "Modbus.lvclass">)  [unwired: 7 in]
                n95 = for {
                  tunnel: w240 -> [w260] mode=indexing
                  shift-right: [w257] -> w235
                  shift-left: w222 -> [w258]
                  shift-right: [w254] -> w236
                  shift-left: w239 -> [w256]
                  n96 = call "parse.vi"("error in (no error)"=w256, "Frame"=w260, "FrameParser in"=refnum<class "DynamicFrameParser.lvclass"> refnum ("RTModbus.lvlib:DynamicFrameParser.lvclass")) -> ("error out"=w255:errorcluster, "FrameParser out"=w259:refnum<class "DynamicFrameParser.lvclass">)  [unwired: 7 in]
                  n97 = call-dynamic "parse.vi"("error in (no error)"=w255, "DynamicFrameParser"=w259, "HPILC in"=w258) -> ("error out"=w254:errorcluster, "ParseSuccessful"=→"ParseSuccessful 4":bool, "HPILC out"=w257:refnum<class "HPILC.lvclass">)  [unwired: 6 in]
                }
                n98 = local write "error out"(w236) -> ()
                n99 = call "getILCData.vi"("ILC in"=w235) -> ("ILCData"=w233:T10, "ILC out"=w234:refnum<class "HPILC.lvclass">)  [unwired: 9 in]
                n100 = Unbundle By Name(w233) -> ("Telemetry"=w232:T5, "Responses"=w231:T4)
                n101 = local write "ILCTelemetry"(w232) -> ()
                n102 = local write "ILCResponses"(w231) -> ()
              }
            }
          }
          event "StepMotor": Value Change {
            n103 = event-data() -> ()  [unwired: 1 in, 6 out]
            n104 = case shown="True" "StepMotor" {
              tunnel: w269 -> [w271 w289]
              tunnel: w268 -> [w270 w307]
              tunnel: [w271 w275] -> w267
              tunnel: [w270 w294] -> w266
              tunnel: w265 -> [_ w304]
              frame False {
              }
              frame True {
                w302 = 0 ("IRQ Number(s)")
                n105 = call "getHPData.vi"("HardPointActuator in"=w289) -> ("HPData"=w293:T14, "HardPointActuator out"=w290:refnum<class "HPILC.lvclass">)  [unwired: 9 in]
                n106 = Bundle By Name(cluster=w293, "Command.Steps"="Steps") -> (w292:T14)
                n107 = call "setHPData.vi"("HPData"=w292, "HardPointActuator in"=w290) -> ("HardPointActuator out"=w288:refnum<class "HPILC.lvclass">)  [unwired: 9 in]
                n108 = call "createStepMotorFrame.vi"("TriggerIRQ"=TRUE, "HardPointActuator in"=w288) -> ("error out"=w285:errorcluster, "Frame"=w286:T9, "HardPointActuator out"=w282:refnum<class "HPILC.lvclass">)  [unwired: 7 in]
                n109 = call-dynamic "addTxBuffer.vi"("error in (no error)"=w285, "Frame"=w286, "Modbus in"=w307) -> ("error out"=w305:errorcluster, "Modbus out"=w306:refnum<class "Modbus.lvclass">)  [unwired: 7 in]
                n110 = call-dynamic "transmit.vi"("error in (no error)"=w305, "Modbus in"=w306) -> ("error out"=w298:errorcluster, "Modbus out"=w295:refnum<class "Modbus.lvclass">)  [unwired: 8 in]
                n111 = xnode "Invoke Method"("FPGA VI Reference In"=w304, "error in"=w298, "IRQ Number(s)"=w302, "Timeout (ms)"=100) -> ("FPGA VI Reference Out"=w303:refnum<k20>, "error out"=w299:errorcluster, "Timed Out"=→"IRQ Timed Out 6":bool)  [unwired: 1 out]
                n112 = xnode "Invoke Method"("FPGA VI Reference In"=w303, "error in"=w299, "IRQ Number(s)"=w302) -> ("error out"=w297:errorcluster)  [unwired: 1 out]
                n113 = flat-sequence {
                  tunnel: w297 -> [w317]
                  tunnel: [w317] -> w296
                  frame #0 {
                    n114 = Wait (ms)(milliseconds to wait=u32 20) -> ()  [unwired: 1 out]
                  }
                }
                n115 = call-dynamic "receive.vi"("error in (no error)"=w296, "Modbus in"=w295) -> ("error out"=w283:errorcluster, "Data"=w284:T9[], "Modbus out"=w294:refnum<class "Modbus.lvclass">)  [unwired: 7 in]
                n116 = for {
                  tunnel: w284 -> [w316] mode=indexing
                  shift-right: [w308] -> w281
                  shift-left: w283 -> [w314]
                  shift-right: [w310] -> w280
                  shift-left: w282 -> [w312]
                  n117 = call "parse.vi"("error in (no error)"=w314, "Frame"=w316, "FrameParser in"=refnum<class "DynamicFrameParser.lvclass"> refnum ("RTModbus.lvlib:DynamicFrameParser.lvclass")) -> ("error out"=w309:errorcluster, "FrameParser out"=w313:refnum<class "DynamicFrameParser.lvclass">)  [unwired: 7 in]
                  n118 = call-dynamic "parse.vi"("error in (no error)"=w309, "DynamicFrameParser"=w313, "HPILC in"=w312) -> ("error out"=w308:errorcluster, "ParseSuccessful"=→"ParseSuccessful 6":bool, "HPILC out"=w310:refnum<class "HPILC.lvclass">)  [unwired: 6 in]
                }
                n119 = call "getHPData.vi"("HardPointActuator in"=w280) -> ("HPData"=w274:T14, "HardPointActuator out"=w279:refnum<class "HPILC.lvclass">)  [unwired: 9 in]
                n120 = local write "error out"(w281) -> ()
                n121 = Unbundle By Name(w274) -> ("Telemetry"=w273:T1, "Responses"=w272:T2)
                n122 = call "getILCData.vi"("ILC in"=w279) -> ("ILCData"=w278:T10, "ILC out"=w275:refnum<class "HPILC.lvclass">)  [unwired: 9 in]
                n123 = Unbundle By Name(w278) -> ("Telemetry"=w277:T5, "Responses"=w276:T4)
                n124 = local write "HPTelemetry"(w273) -> ()
                n125 = local write "HPResponses"(w272) -> ()
                n126 = local write "ILCTelemetry"(w277) -> ()
                n127 = local write "ILCResponses"(w276) -> ()
              }
            }
          }
          event "ForceAndStatus": Value Change {
            n128 = event-data() -> ()  [unwired: 1 in, 6 out]
            n129 = case shown="True" "ForceAndStatus" {
              tunnel: w324 -> [w326 w330]
              tunnel: w323 -> [w325 w357]
              tunnel: [w326 w335] -> w322
              tunnel: [w325 w344] -> w321
              tunnel: w320 -> [_ w354]
              frame False {
              }
              frame True {
                w352 = 0 ("IRQ Number(s)")
                n130 = call "createForceAndStatusFrame.vi"("TriggerIRQ"=TRUE, "HardPointActuator in"=w330) -> ("error out"=w327:errorcluster, "Frame"=w328:T9, "HardPointActuator out"=w329:refnum<class "HPILC.lvclass">)  [unwired: 7 in]
                n131 = call-dynamic "addTxBuffer.vi"("error in (no error)"=w327, "Frame"=w328, "Modbus in"=w357) -> ("error out"=w355:errorcluster, "Modbus out"=w356:refnum<class "Modbus.lvclass">)  [unwired: 7 in]
                n132 = call-dynamic "transmit.vi"("error in (no error)"=w355, "Modbus in"=w356) -> ("error out"=w348:errorcluster, "Modbus out"=w345:refnum<class "Modbus.lvclass">)  [unwired: 8 in]
                n133 = xnode "Invoke Method"("FPGA VI Reference In"=w354, "error in"=w348, "IRQ Number(s)"=w352, "Timeout (ms)"=100) -> ("FPGA VI Reference Out"=w353:refnum<k20>, "error out"=w349:errorcluster, "Timed Out"=→"IRQ Timed Out 7":bool)  [unwired: 1 out]
                n134 = xnode "Invoke Method"("FPGA VI Reference In"=w353, "error in"=w349, "IRQ Number(s)"=w352) -> ("error out"=w347:errorcluster)  [unwired: 1 out]
                n135 = flat-sequence {
                  tunnel: w347 -> [w367]
                  tunnel: [w367] -> w346
                  frame #0 {
                    n136 = Wait (ms)(milliseconds to wait=u32 20) -> ()  [unwired: 1 out]
                  }
                }
                n137 = call-dynamic "receive.vi"("error in (no error)"=w346, "Modbus in"=w345) -> ("error out"=w342:errorcluster, "Data"=w343:T9[], "Modbus out"=w344:refnum<class "Modbus.lvclass">)  [unwired: 7 in]
                n138 = for {
                  tunnel: w343 -> [w366] mode=indexing
                  shift-right: [w358] -> w341
                  shift-left: w342 -> [w364]
                  shift-right: [w360] -> w340
                  shift-left: w329 -> [w362]
                  n139 = call "parse.vi"("error in (no error)"=w364, "Frame"=w366, "FrameParser in"=refnum<class "DynamicFrameParser.lvclass"> refnum ("RTModbus.lvlib:DynamicFrameParser.lvclass")) -> ("error out"=w359:errorcluster, "FrameParser out"=w363:refnum<class "DynamicFrameParser.lvclass">)  [unwired: 7 in]
                  n140 = call-dynamic "parse.vi"("error in (no error)"=w359, "DynamicFrameParser"=w363, "HPILC in"=w362) -> ("error out"=w358:errorcluster, "ParseSuccessful"=→"ParseSuccessful 7":bool, "HPILC out"=w360:refnum<class "HPILC.lvclass">)  [unwired: 6 in]
                }
                n141 = call "getHPData.vi"("HardPointActuator in"=w340) -> ("HPData"=w334:T14, "HardPointActuator out"=w339:refnum<class "HPILC.lvclass">)  [unwired: 9 in]
                n142 = local write "error out"(w341) -> ()
                n143 = Unbundle By Name(w334) -> ("Telemetry"=w333:T1, "Responses"=w332:T2)
                n144 = call "getILCData.vi"("ILC in"=w339) -> ("ILCData"=w338:T10, "ILC out"=w335:refnum<class "HPILC.lvclass">)  [unwired: 9 in]
                n145 = Unbundle By Name(w338) -> ("Telemetry"=w337:T5, "Responses"=w336:T4)
                n146 = local write "HPTelemetry"(w333) -> ()
                n147 = local write "HPResponses"(w332) -> ()
                n148 = local write "ILCTelemetry"(w337) -> ()
                n149 = local write "ILCResponses"(w336) -> ()
              }
            }
          }
          event "Reset": Value Change {
            n150 = event-data() -> ()  [unwired: 1 in, 6 out]
            n151 = case shown="True" "Reset" {
              tunnel: w374 -> [w376 w377]
              tunnel: w373 -> [w375 w403]
              tunnel: [w376 w385] -> w372
              tunnel: [w375 w388] -> w371
              tunnel: w370 -> [_ w400]
              frame False {
              }
              frame True {
                w398 = 0 ("IRQ Number(s)")
                n152 = call "createResetFrame.vi"("TriggerIRQ"=TRUE, "ILC in"=w377) -> ("error out"=w381:errorcluster, "Frame"=w380:T9, "ILC out"=w379:refnum<class "HPILC.lvclass">)  [unwired: 7 in]
                n153 = call-dynamic "addTxBuffer.vi"("error in (no error)"=w381, "Frame"=w380, "Modbus in"=w403) -> ("error out"=w401:errorcluster, "Modbus out"=w402:refnum<class "Modbus.lvclass">)  [unwired: 7 in]
                n154 = call-dynamic "transmit.vi"("error in (no error)"=w401, "Modbus in"=w402) -> ("error out"=w394:errorcluster, "Modbus out"=w389:refnum<class "Modbus.lvclass">)  [unwired: 8 in]
                n155 = xnode "Invoke Method"("FPGA VI Reference In"=w400, "error in"=w394, "IRQ Number(s)"=w398, "Timeout (ms)"=100) -> ("FPGA VI Reference Out"=w399:refnum<k20>, "error out"=w395:errorcluster, "Timed Out"=→"IRQ Timed Out 5":bool)  [unwired: 1 out]
                n156 = xnode "Invoke Method"("FPGA VI Reference In"=w399, "error in"=w395, "IRQ Number(s)"=w398) -> ("error out"=w393:errorcluster)  [unwired: 1 out]
                n157 = flat-sequence {
                  tunnel: w393 -> [w413]
                  tunnel: [w413] -> w392
                  frame #0 {
                    n158 = Wait (ms)(milliseconds to wait=u32 20) -> ()  [unwired: 1 out]
                  }
                }
                n159 = call-dynamic "receive.vi"("error in (no error)"=w392, "Modbus in"=w389) -> ("error out"=w390:errorcluster, "Data"=w391:T9[], "Modbus out"=w388:refnum<class "Modbus.lvclass">)  [unwired: 7 in]
                n160 = for {
                  tunnel: w391 -> [w411] mode=indexing
                  shift-right: [w408] -> w386
                  shift-left: w379 -> [w409]
                  shift-right: [w405] -> w387
                  shift-left: w390 -> [w407]
                  n161 = call "parse.vi"("error in (no error)"=w407, "Frame"=w411, "FrameParser in"=refnum<class "DynamicFrameParser.lvclass"> refnum ("RTModbus.lvlib:DynamicFrameParser.lvclass")) -> ("error out"=w406:errorcluster, "FrameParser out"=w410:refnum<class "DynamicFrameParser.lvclass">)  [unwired: 7 in]
                  n162 = call-dynamic "parse.vi"("error in (no error)"=w406, "DynamicFrameParser"=w410, "HPILC in"=w409) -> ("error out"=w405:errorcluster, "ParseSuccessful"=→"ParseSuccessful 5":bool, "HPILC out"=w408:refnum<class "HPILC.lvclass">)  [unwired: 6 in]
                }
                n163 = local write "error out"(w387) -> ()
                n164 = call "getILCData.vi"("ILC in"=w386) -> ("ILCData"=w384:T10, "ILC out"=w385:refnum<class "HPILC.lvclass">)  [unwired: 9 in]
                n165 = Unbundle By Name(w384) -> ("Telemetry"=w383:T5, "Responses"=w382:T4)
                n166 = local write "ILCTelemetry"(w383) -> ()
                n167 = local write "ILCResponses"(w382) -> ()
              }
            }
          }
        }
      }
    }
    frame #3 {
      n168 = xnode "Invoke Method"("FPGA VI Reference In"=w415) -> ("FPGA VI Reference Out"=w416:refnum<k20>)  [unwired: 1 in, 1 out]
      n169 = xnode "Close FPGA VI Reference"("FPGA VI Reference In"=w416) -> ()  [unwired: 1 in, 1 out]
    }
  }
